vi "Get Required Driver Types.vi"(8 "error in (no error)":errorcluster, 11 "Test Multi Instrument Msg in":refnum<class "Test Multi Instrument Msg.lvclass">) -> (0 "error out":errorcluster, 2 "Required Driver Types":T1[](array[typedef]), 3 "Test Multi Instrument Msg out":refnum<class "Test Multi Instrument Msg.lvclass">)   [LabVIEW 2020, in "Test.lvlib" / "Test Multi Instrument Msg.lvclass"]
doc: "Get the Required Driver Types and count of each driver for execution of the Instrument Msg."
uses:
  Test Multi Instrument Msg.lvclass
  PPL/HDH.Actor Framework.Core.Instrument Handler.lvlibp/Messages/Multi Instrument Msg/Ctl_RequiredInstrumentElement.ctl
  PPL/HDH.Actor Framework.Core.Instrument Driver.lvlibp/Instrument Driver/Instrument Driver.lvclass
  Instrument/Test Instrument/Test Instrument.lvclass
  C:/Current projects/WS/PPL/HDH.Actor Framework.Core.Instrument Driver.lvlibp/Instrument Driver/Instrument Driver.lvclass
  PPL/HDH.Actor Framework.Core.Instrument Handler.lvlibp/Messages/Multi Instrument Msg/Multi Instrument Msg.lvclass
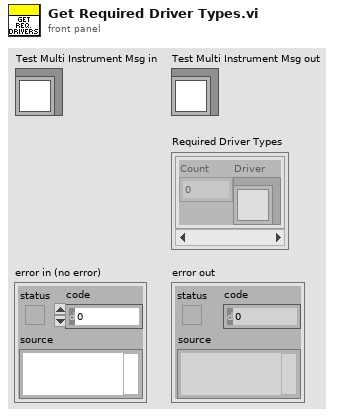
[diagram p1: front panel]
types:
  T1 = typedef "HDH.Actor Framework.Core.Instrument Handler.lvlibp/Multi Instrument Msg.lvclass/Ctl_RequiredInstrumentElement.ctl" = cluster{"Count":i16, "Driver":refnum<class "Instrument Driver.lvclass">}
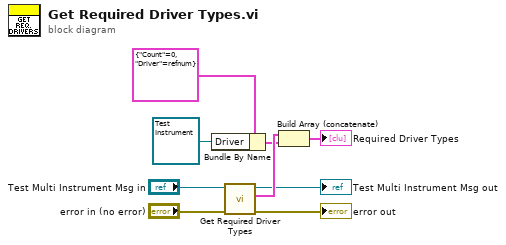
[diagram p0: block diagram]
diagram:
  n1 = Bundle By Name(cluster=T1 {"Count"=0, "Driver"=refnum} ("Required Driver Types"), "Driver"=refnum<class "Test Instrument.lvclass"> refnum ("Test.lvlib:Test Instrument.lvclass")) -> (w1:T1)
  n2 = call-parent "Get Required Driver Types.vi"("error in (no error)"="error in (no error)", "Multi Instrument Msg in"="Test Multi Instrument Msg in") -> ("error out"=→"error out":errorcluster, "Required Driver Types"=w8:T1[], "Multi Instrument Msg out"=→"Test Multi Instrument Msg out":refnum<class "Test Multi Instrument Msg.lvclass">)  [unwired: 7 in]
  n3 = Build Array (concatenate)(w8, w1) -> (→"Required Driver Types":T1[])
